vi "SplineHelp_GetCubicCtrlVectorsFromWeightedWayPts.vi"(9 "Use Weights":bool, 11 "WeightedWayPoints":T1[](array[typedef]) {"SCALAR" format="%14.3f"; "ROTATION"."SIN" format="%13.4f"; "ROTATION"."COS" format="%13.4f"; "ROTATION"."VALUE" format="%13.4f"; "TRANSLATION"."Y" format="%14.3f"; "TRANSLATION"."X" format="%14.3f"}) -> (1 "Interior WAYPOINTS":T2[](array[typedef]) {"Y" format="%14.3f"; "X" format="%14.3f"}, 3 "SplineControlVectors":T4[](array[typedef]))   [LabVIEW 2019, in "Trajectory_Library.lvlib"]
doc: "Returns 2 cubic control vectors from a set of exterior weighted waypoints and interior translations.\n\nParameters: \n - startWayPoint - The starting weighted waypoint.\n - interiorWaypoints - The interior waypoints (Translation).\n - endWayPoint - The ending weighted waypoint\n\nReturns:\n - SplineControlVectors - Array of cubic control vectors."
uses:
  Trajectory_Library.lvlib
  WEIGHTED_WAYPOINT.ctl
  TRANSLATION2D.ctl
  ROTATION2D.ctl
  SPLINE_CTRL_VECTOR.ctl
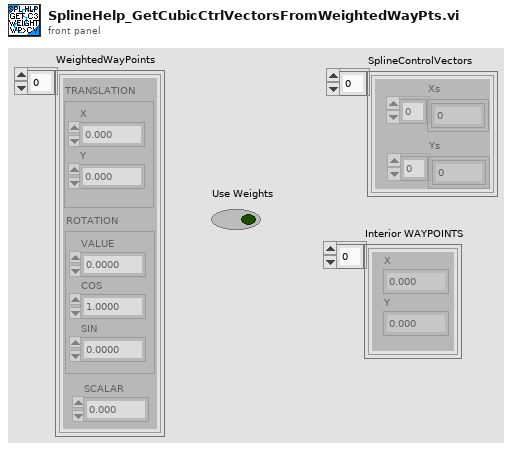
[diagram p1: front panel]
types:
  T1 = typedef "Trajectory_Library.lvlib/WEIGHTED_WAYPOINT.ctl" = cluster{"TRANSLATION":T2, "ROTATION":T3, "SCALAR":dbl}
  T2 = typedef "Trajectory_Library.lvlib/TRANSLATION2D.ctl" = cluster{"X":dbl, "Y":dbl}
  T3 = typedef "Trajectory_Library.lvlib/ROTATION2D.ctl" = cluster{"VALUE":dbl, "COS":dbl, "SIN":dbl}
  T4 = typedef "Trajectory_Library.lvlib/SPLINE_CTRL_VECTOR.ctl" = cluster{"Xs":dbl[], "Ys":dbl[]}
  T5 = typedef "Trajectory_Library.lvlib/POSE2D.ctl" = cluster{"TRANSLATION":T2, "ROTATION":T3}
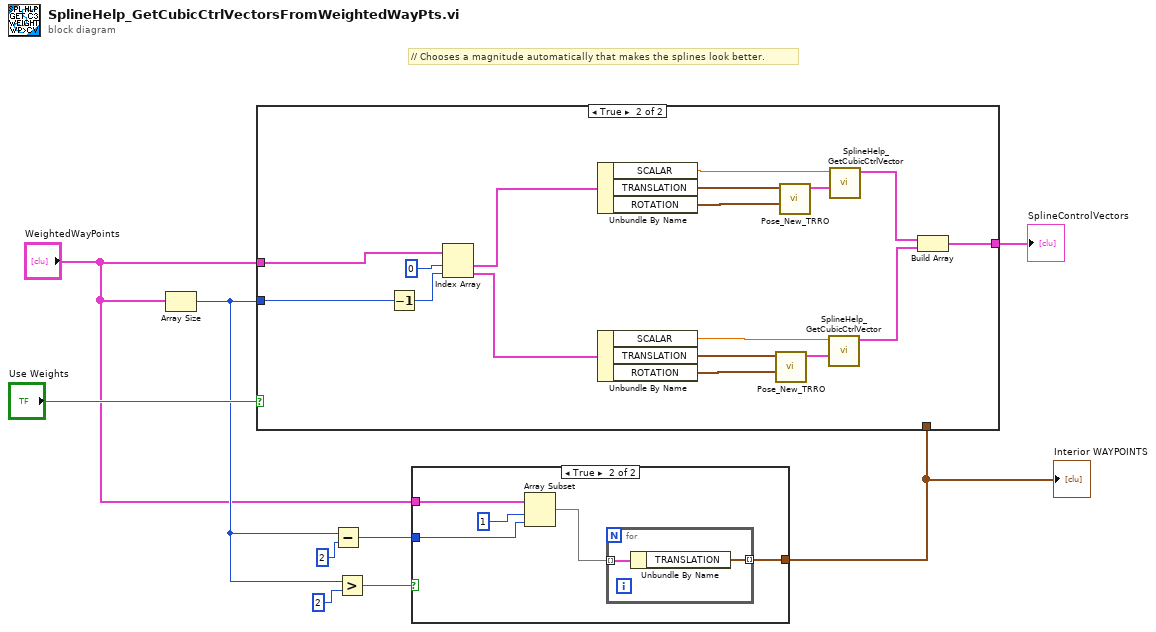
[diagram p0: block diagram]
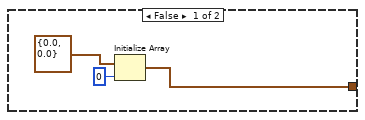
[diagram p2: hidden frame]
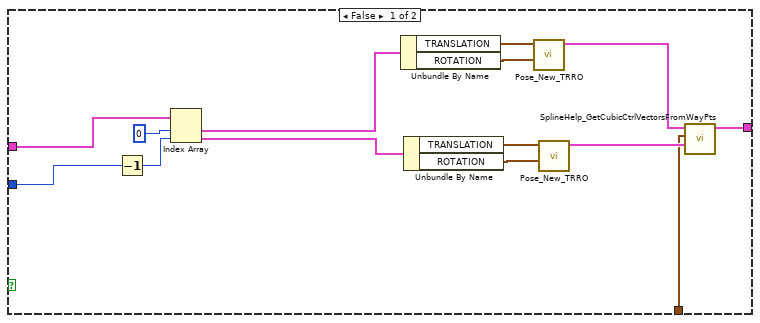
[diagram p3: hidden frame]
diagram:
  # "// Chooses a magnitude automatically that makes the splines look better."
  n1 = Array Size(array="WeightedWayPoints") -> (size(s)=w7:i32)
  n2 = Subtract(x=w7, y=2) -> (x-y=w6:i32)
  n3 = Greater?(x=w7, y=2) -> (0:w5:bool)
  n4 = case shown="True" w5 {
    tunnel: [w10 w17] -> w1
    tunnel: "WeightedWayPoints" -> [_ w16]
    tunnel: w6 -> [_ w14]
    frame False {
      n5 = Initialize Array(T2 {"X"=0.0, "Y"=0.0} ("TRANSLATION"), 0 ("dimension size")) -> (w10:T2[])
    }
    frame True {
      n6 = Array Subset(array=w16, index=1, length=w14) -> (w13:T1[])
      n7 = for {
        tunnel: [w18] -> w17 mode=indexing
        tunnel: w13 -> [w19] mode=indexing
        n8 = Unbundle By Name(w19) -> ("TRANSLATION"=w18:T2)
      }
    }
  }
  "Interior WAYPOINTS" <- w1
  n9 = case shown="True" "Use Weights" {
    tunnel: [w33 w48] -> w9
    tunnel: "WeightedWayPoints" -> [w24 w43]
    tunnel: w7 -> [w21 w42]
    tunnel: w1 -> [w20 _]
    frame False {
      n10 = Decrement(x=w21) -> (x-1=w25:i32)
      n11 = Index Array(array=w24, index #1=0 ("index"), index #2=w25) -> (element #1=w23:T1, element #2=w22:T1)
      n12 = Unbundle By Name(w23) -> ("TRANSLATION"=w30:T2, "ROTATION"=w29:T3)
      n13 = Unbundle By Name(w22) -> ("TRANSLATION"=w32:T2, "ROTATION"=w31:T3)
      n14 = call "Pose_New_TRRO.vi"("ROTATION"=w29, "TRANSLATION"=w30) -> ("outPOSE"=w27:T5)  [unwired: 9 in]
      n15 = call "Pose_New_TRRO.vi"("ROTATION"=w31, "TRANSLATION"=w32) -> ("outPOSE"=w28:T5)  [unwired: 9 in]
      n16 = call "SplineHelp_GetCubicCtrlVectorsFromWayPts.vi"("Enging POSE"=w28, "Interior WAYPOINTS"=w20, "Starting POSE"=w27) -> ("SplineControlVectors"=w33:T4[])  [unwired: 8 in]
    }
    frame True {
      n17 = Decrement(x=w42) -> (x-1=w44:i32)
      n18 = Index Array(array=w43, index #1=0 ("index"), index #2=w44) -> (element #1=w41:T1, element #2=w40:T1)
      n19 = Unbundle By Name(w41) -> ("SCALAR"=w37:dbl, "TRANSLATION"=w38:T2, "ROTATION"=w39:T3)
      n20 = Unbundle By Name(w40) -> ("SCALAR"=w34:dbl, "TRANSLATION"=w35:T2, "ROTATION"=w36:T3)
      n21 = call "Pose_New_TRRO.vi"("ROTATION"=w36, "TRANSLATION"=w35) -> ("outPOSE"=w47:T5)  [unwired: 9 in]
      n22 = call "Pose_New_TRRO.vi"("ROTATION"=w39, "TRANSLATION"=w38) -> ("outPOSE"=w46:T5)  [unwired: 9 in]
      n23 = call "SplineHelp_GetCubicCtrlVector.vi"("Input POSE"=w47, "Scalar"=w34) -> ("resultSpline_Ctrl_Vector"=w49:T4)  [unwired: 9 in]
      n24 = call "SplineHelp_GetCubicCtrlVector.vi"("Input POSE"=w46, "Scalar"=w37) -> ("resultSpline_Ctrl_Vector"=w50:T4)  [unwired: 9 in]
      n25 = Build Array(w50, w49) -> (w48:T4[])
    }
  }
  "SplineControlVectors" <- w9
